vi "Sistema de ventilación_V0.vi"() -> ()   [LabVIEW 2023]
uses:
  <vilib>/MakerHub/LINX/Public/Peripherals/Analog/Analog Read 1 Chan.vi
  <vilib>/MakerHub/LINX/Public/Peripherals/Digital/Digital Write 1 Chan.vi
  <vilib>/MakerHub/LINX/Public/Peripherals/Analog/Analog Read N Chans.vi
  <vilib>/MakerHub/LINX/Public/Peripherals/Digital/Digital Write N Chans.vi
  <vilib>/MakerHub/LINX/Private/Local IO/LinxAnalogRead.vi
  <vilib>/MakerHub/LINX/Public/Utilities/Check Channel.vi
  <vilib>/MakerHub/LINX/Private/Local IO/LinxDigitalWrite.vi
  <vilib>/MakerHub/LINX/Public/Utilities/Open Serial.vi
  <vilib>/MakerHub/LINX/Public/Sensors/Motion/Servo/Servo Open One Channel.vi
  <vilib>/MakerHub/LINX/Public/Peripherals/Analog/Analog Write 1 Chan.vi
  <vilib>/MakerHub/LINX/Private/Utilties/Generate Error.vi
  <vilib>/MakerHub/LINX/Public/Sensors/Temperature/TMP3x/TMP35.vi
  <vilib>/MakerHub/LINX/Public/Sensors/Motion/Servo/Servo Set Pulse Width One Channel.vi
  <vilib>/MakerHub/LINX/Public/Sensors/Motion/Servo/Servo Close One Channel.vi
  <vilib>/MakerHub/LINX/LMH-LINX.lvlib
  <vilib>/MakerHub/LINX/Public/Sensors/Temperature/TMP3x/TMP3x.lvlib
  <vilib>/MakerHub/LINX/Public/Sensors/Motion/Servo/Servo.lvlib
panel:
  out "?":bool
  out "?":bool
  out "?":bool
  out "?":bool
  in  "?":bool
  out "Serevo Aire Angulo":string
  out "Serevo Temp Angulo":string
  in  "Serial Port":refnum<visa-resource-name>
  out "?":bool
  out "?":bool
  out "?":bool
  out "?":bool
  out "?":bool
  out "?":bool
  out "?":bool
  out "?":bool
  out "?":bool
  out "?":bool
  out "?":bool
  out "?":bool
  out "?":bool
  out "?":bool
  out "?":bool
  out "?":bool
  out "?":bool
  out "?":bool
  in  "?":bool
  out "Filtro de Calor":bool
  out "Filtro de Aire":bool
  out "Calidad del aire":dbl(knob) scale=0.0..1800.0
  out "Temperatura":dbl(slide) scale=0.0..60.0
  out "t [sec]":dbl
  out "Iteration No":i32
  in  "?":bool
  out "VI is running?":bool caption="ON/OFF"
  # "SISTEMA DE VENTILACIÓN DE DOBLE FLUJO"
  # "Entrada"
  # "Salida"
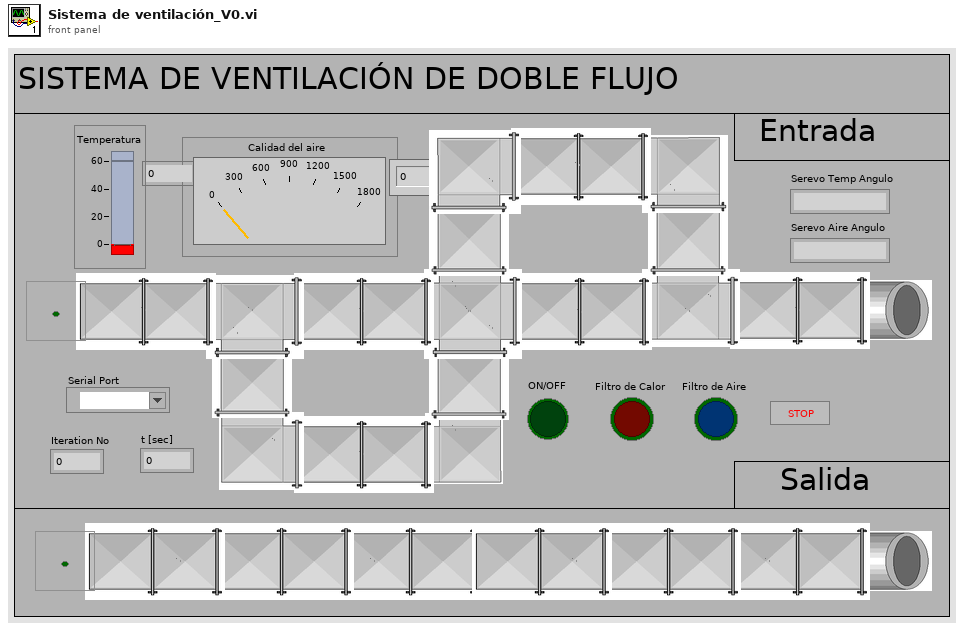
[diagram p1: front panel]
types:
  T1 = typedef "LMH-LINX.lvlib/LINX Ref.ctl" = cluster{"IO":T2, "Interface":T3, "LINX Device Config":T4}
  T2 = typedef "LMH-LINX.lvlib/Platform.ctl" = enum16{"Remote", "Local"}
  T3 = typedef "LMH-LINX.lvlib/Interface.ctl" = enum16{"Serial", "TCP"}
  T4 = typedef "LMH-LINX.lvlib/Device.lvlib/LINX Device Config.ctl" = cluster{"Interface":T3, "COM Port":refnum<visa-resource-name>, "TCP Configuration":T5, "Device Family":u8, "Device ID":u8, "Device Name":string, "TCP Ref":refnum<k5>, "Channels":T6}
  T5 = typedef "LMH-LINX.lvlib/Device.lvlib/TCP Config.ctl" = cluster{"IP Address":string, "Port":u16}
  T6 = typedef "LMH-LINX.lvlib/Channels.ctl" = cluster{"DI":u8[], "DO":u8[], "AI":u8[], "AO":u8[], "PWM":u8[], "QE":u8[], "UART":u8[], "I2C 2":u8[], "SPI":u8[], "CAN":u8[], "Servo":u8[], "AI Ref (V)":dbl, "AI Resolution (Bits)":u8, "AO Ref (V)":dbl, "AO Resolution (Bits)":u8}
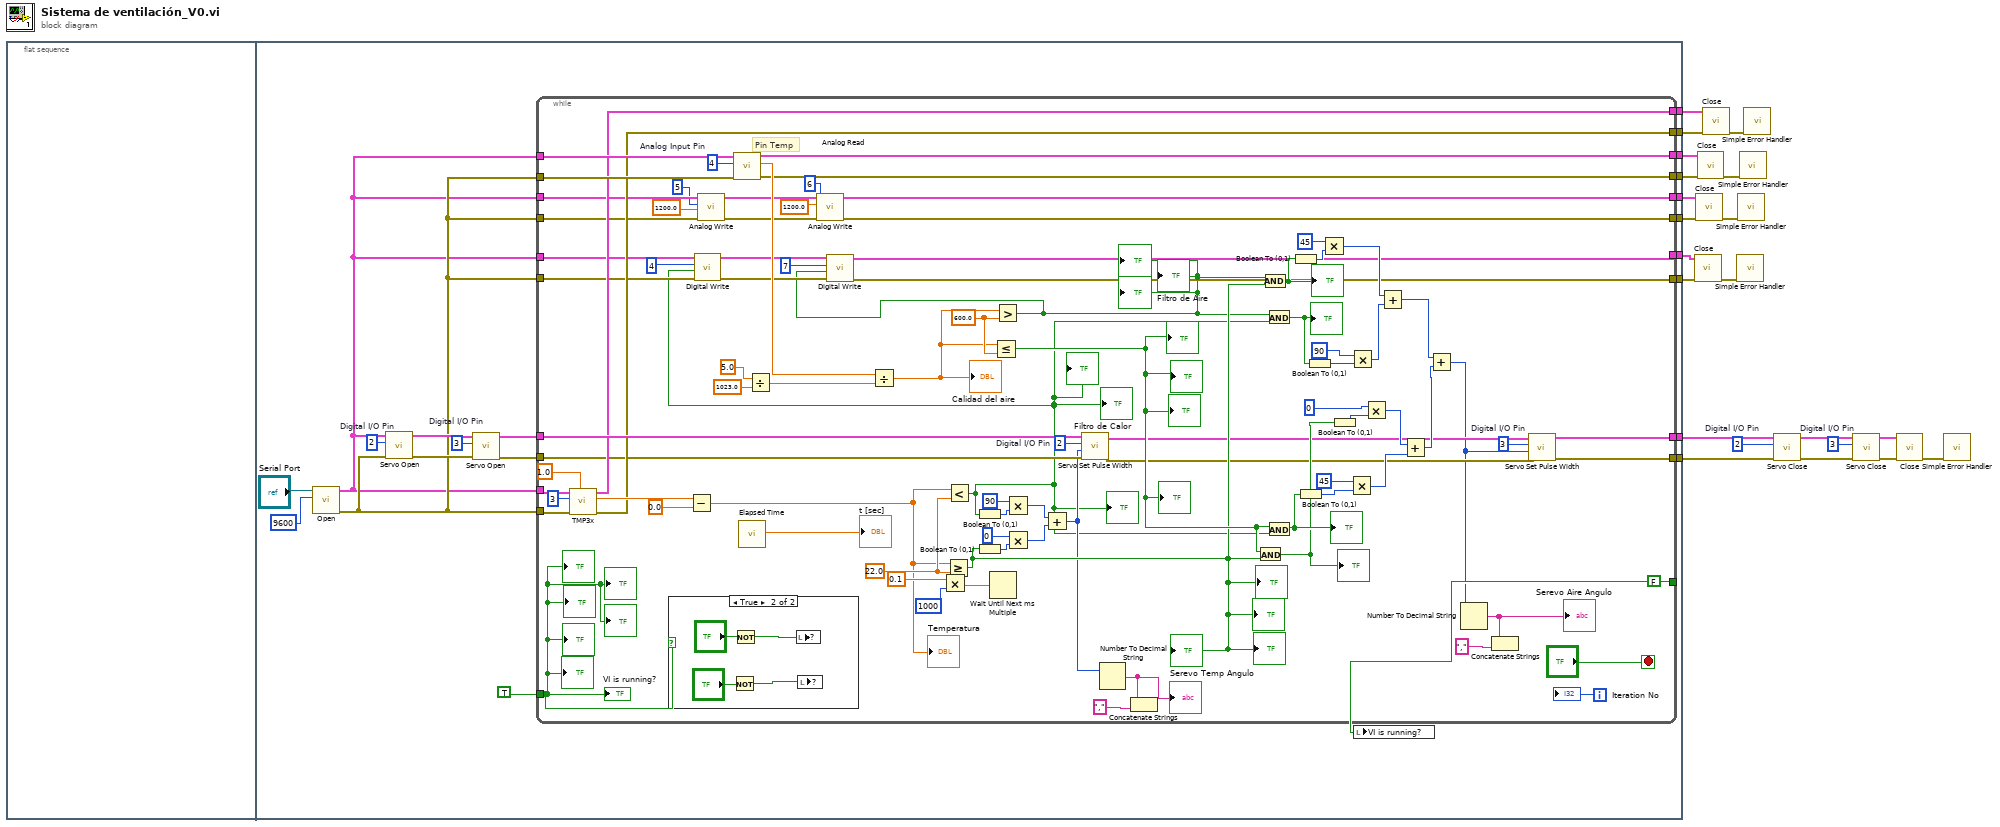
[diagram p0: block diagram]
diagram:
  w12 = 3  # Digital I/O Pin
  w13 = 2  # Digital I/O Pin
  n1 = flat-sequence {
    tunnel: [w40] -> w21
    tunnel: [w38] -> w19
    tunnel: [w37] -> w17
    tunnel: [w36] -> w16
    tunnel: [w35] -> w15
    tunnel: [w34] -> w14
    tunnel: [w27] -> w5
    tunnel: [w26] -> w4
    tunnel: [w23] -> w2
    tunnel: [w22] -> w1
    frame #0 {
    }
    frame #1 {
      w32 = 3  # Digital I/O Pin
      w33 = 2  # Digital I/O Pin
      n2 = call-poly <vilib>:"Open.vi"("Baud Rate Override"=u32 9600, "Serial Port"="Serial Port") -> ("Error Out"=w25:errorcluster, "LINX Resource"=w24:T1)  [unwired: 7 in, 1 out]
      n3 = call-poly <vilib>:"Servo Open.vi"("Error In"=w25, "Servo Channel"=w33, "LINX Resource"=w24) -> ("Error Out"=w31:errorcluster, "LINX Resource"=w29:T1)  [unwired: 7 in]
      n4 = call-poly <vilib>:"Servo Open.vi"("Error In"=w31, "Servo Channel"=w32, "LINX Resource"=w29) -> ("Error Out"=w30:errorcluster, "LINX Resource"=w28:T1)  [unwired: 7 in]
      n5 = while {
        tunnel: [FALSE] -> w42
        tunnel: TRUE -> [w54]
        tunnel: w24 -> [w123]
        tunnel: [w80] -> w40
        tunnel: w25 -> [w121]
        tunnel: w24 -> [w116]
        tunnel: [w81] -> w38
        tunnel: w25 -> [w110]
        tunnel: [w74] -> w37
        tunnel: [w73] -> w36
        tunnel: w28 -> [w82]
        tunnel: w30 -> [w79]
        tunnel: [w76] -> w35
        tunnel: [w75] -> w34
        tunnel: w25 -> [w70]
        tunnel: w24 -> [w69]
        tunnel: [w62] -> w27
        tunnel: [w61] -> w26
        tunnel: w25 -> [w53]
        tunnel: w24 -> [w52]
        tunnel: [w47] -> w23
        tunnel: [w46] -> w22
        i -> [w127]
        stop <- "?" stop-if-true
        w78 = 2  # Digital I/O Pin
        w71 = 3  # Digital I/O Pin
        w109 = 4  # Analog Input Pin
        w125 = 600.0
        w124 = 22.0
        # "Pin Temp"
        n6 = call-poly <vilib>:"TMP3x.vi"("Analog Ref Override"=1.0, "Error In"=w121, "Analog Channel"=3, "LINX Resource"=w123) -> ("Error Out"=w81:errorcluster, "Temp C"=w119:dbl, "LINX Resource"=w80:T1)  [unwired: 5 in]
        n7 = case shown="True" w54 {
          frame False {
          }
          frame True {
            n8 = Not(x="?") -> (.not. x?=w133:bool)
            n9 = Not(x="?") -> (.not. x?=w135:bool)
            n10 = local write item#8(w135) -> ()
            n11 = local write item#30(w133) -> ()
          }
        }
        n12 = Subtract(x=w119, y=0.0) -> (x-y=w118:dbl)
        "Temperatura" <- w118
        n13 = call-poly <vilib>:"Analog Write.vi"("Error In"=w70, "AO Value"=1200.0, "AO Channel"=5, "LINX Resource"=w69) -> ("Error Out"=w63:errorcluster, "LINX Resource"=w64:T1)  [unwired: 6 in]
        n14 = call-poly <vilib>:"Analog Read.vi"("Error In"=w110, "Analog Channel"=w109, "LINX Resource"=w116) -> ("Error Out"=w73:errorcluster, "Voltage"=w113:dbl, "LINX Resource"=w74:T1)  [unwired: 5 in, 1 out]
        n15 = call "Elapsed Time"() -> ("Elapsed Time (s)"=→"t [sec]":dbl)  [unwired: 12 in, 7 out]
        n16 = Divide(x=5.0, y=1023.0) -> (x/y=w112:dbl)
        n17 = call-poly <vilib>:"Analog Write.vi"("Error In"=w63, "AO Value"=1200.0, "AO Channel"=6, "LINX Resource"=w64) -> ("Error Out"=w62:errorcluster, "LINX Resource"=w61:T1)  [unwired: 6 in]
        n18 = Divide(x=w113, y=w112) -> (x/y=w111:dbl)
        "Calidad del aire" <- w111
        n19 = Multiply(x=0.1, y=1000) -> (x*y=w130:dbl)
        n20 = Greater Or Equal?(x=w118, y=w124) -> (x >= y?=w85:bool)
        "?" <- w85
        "?" <- w85
        "?" <- w85
        "?" <- w85
        n21 = Less?(x=w118, y=w124) -> (x < y?=w45:bool)
        "Filtro de Calor" <- w45
        "?" <- w45
        "?" <- w45
        n22 = call-poly <vilib>:"Digital Write.vi"("Error In"=w53, "Output Value"=w45, "DO Channel"=4, "LINX Resource"=w52) -> ("Error Out"=w48:errorcluster, "LINX Resource"=w49:T1)  [unwired: 6 in]
        n23 = Boolean To (0,1)(Boolean=w45) -> (0, 1=w88:i16)
        n24 = Boolean To (0,1)(Boolean=w85) -> (0, 1=w86:i16)
        n25 = Wait Until Next ms Multiple(millisecond multiple=w130) -> ()  [unwired: 1 out]
        n26 = Less Or Equal?(x=w111, y=w125) -> (x <= y?=w117:bool)
        "?" <- w117
        "?" <- w117
        "?" <- w117
        "?" <- w117
        n27 = Greater?(x=w111, y=w125) -> (0:w44:bool)
        "Filtro de Aire" <- w44
        "?" <- w44
        "?" <- w44
        n28 = call-poly <vilib>:"Digital Write.vi"("Error In"=w48, "Output Value"=w44, "DO Channel"=7, "LINX Resource"=w49) -> ("Error Out"=w46:errorcluster, "LINX Resource"=w47:T1)  [unwired: 6 in]
        n29 = Multiply(x=90, y=w88) -> (x*y=w83:i32)
        n30 = Multiply(x=0, y=w86) -> (x*y=w84:i32)
        n31 = Add(x=w83, y=w84) -> (x+y=w58:i32)
        n32 = call-poly <vilib>:"Servo Set Pulse Width.vi"("Error In"=w79, "Pulse Width (uS)"=w58, "Servo Channel"=w78, "LINX Resource"=w82) -> ("Error Out"=w77:errorcluster, "LINX Resource"=w72:T1)  [unwired: 6 in]
        n33 = Number To Decimal String(number=w58) -> (decimal integer string=w60:string)  [unwired: 1 in]
        "Serevo Temp Angulo" <- w60
        n34 = Concatenate Strings(w60, "," ("string")) -> ()  [unwired: 1 out]
        n35 = And(x=w117, y=w85) -> (x .and. y?=w99:bool)
        "?" <- w99
        n36 = And(x=w44, y=w85) -> (x .and. y?=w106:bool)
        "?" <- w106
        n37 = And(x=w44, y=w45) -> (x .and. y?=w96:bool)
        "?" <- w96
        n38 = And(x=w117, y=w45) -> (x .and. y?=w102:bool)
        "?" <- w102
        n39 = Boolean To (0,1)(Boolean=w106) -> (0, 1=w105:i16)
        n40 = Boolean To (0,1)(Boolean=w102) -> (0, 1=w103:i16)
        n41 = Boolean To (0,1)(Boolean=w96) -> (0, 1=w97:i16)
        n42 = Multiply(x=45, y=w105) -> (x*y=w95:i32)
        n43 = Boolean To (0,1)(Boolean=w99) -> (0, 1=w100:i16)
        n44 = Multiply(x=45, y=w103) -> (x*y=w92:i32)
        n45 = Multiply(x=90, y=w97) -> (x*y=w94:i32)
        n46 = Multiply(x=0, y=w100) -> (x*y=w93:i32)
        n47 = Add(x=w95, y=w94) -> (x+y=w90:i32)
        n48 = Add(x=w92, y=w93) -> (x+y=w91:i32)
        n49 = Add(x=w90, y=w91) -> (x+y=w55:i32)
        n50 = Number To Decimal String(number=w55) -> (decimal integer string=w57:string)  [unwired: 1 in]
        "Serevo Aire Angulo" <- w57
        n51 = Concatenate Strings(w57, "," ("string")) -> ()  [unwired: 1 out]
        n52 = call-poly <vilib>:"Servo Set Pulse Width.vi"("Error In"=w77, "Pulse Width (uS)"=w55, "Servo Channel"=w71, "LINX Resource"=w72) -> ("Error Out"=w75:errorcluster, "LINX Resource"=w76:T1)  [unwired: 6 in]
        "VI is running?" <- w54
        "Iteration No" <- w127
        "?" <- w54
        "?" <- w54
        "?" <- w54
        "?" <- w54
        "?" <- w54
        "?" <- w54
      }
      n53 = local write "VI is running?"(w42) -> ()
    }
  }
  n54 = call <vilib>:"Close.vi"("Error In"=w1, "LINX Resource"=w2) -> ("Error Out"=w3:errorcluster)  [unwired: 9 in]
  n55 = call <vilib>:"Close.vi"("Error In"=w5, "LINX Resource"=w4) -> ("Error Out"=w6:errorcluster)  [unwired: 9 in]
  n56 = call <vilib>:"Close.vi"("Error In"=w16, "LINX Resource"=w17) -> ("Error Out"=w18:errorcluster)  [unwired: 9 in]
  n57 = call <vilib>:"Close.vi"("Error In"=w19, "LINX Resource"=w21) -> ("Error Out"=w20:errorcluster)  [unwired: 9 in]
  n58 = call <vilib>:"Simple Error Handler.vi"("error in (no error)"=w3) -> ()  [unwired: 4 in, 5 out]
  n59 = call <vilib>:"Simple Error Handler.vi"("error in (no error)"=w6) -> ()  [unwired: 4 in, 5 out]
  n60 = call <vilib>:"Simple Error Handler.vi"("error in (no error)"=w18) -> ()  [unwired: 4 in, 5 out]
  n61 = call <vilib>:"Simple Error Handler.vi"("error in (no error)"=w20) -> ()  [unwired: 4 in, 5 out]
  n62 = call-poly <vilib>:"Servo Close.vi"("Error In"=w14, "Servo Channel"=w13, "LINX Resource"=w15) -> ("Error Out"=w9:errorcluster, "LINX Resource"=w11:T1)  [unwired: 7 in]
  n63 = call-poly <vilib>:"Servo Close.vi"("Error In"=w9, "Servo Channel"=w12, "LINX Resource"=w11) -> ("Error Out"=w8:errorcluster, "LINX Resource"=w10:T1)  [unwired: 7 in]
  n64 = call <vilib>:"Close.vi"("Error In"=w8, "LINX Resource"=w10) -> ("Error Out"=w7:errorcluster)  [unwired: 9 in]
  n65 = call <vilib>:"Simple Error Handler.vi"("error in (no error)"=w7) -> ()  [unwired: 4 in, 5 out]
